vi "Extract core 2D array.vi"(8 "error in (no error)":errorcluster, 10 "Core extraction size":i32=25, 11 "Image Pixels (I16)":i16[][](array[numeric])=array512x512[262144 elements]) -> (0 "error out":errorcluster, 3 "subarray":i16[][](array[numeric]))   [LabVIEW 2020]
panel:
  out "dim2_length":i32
  out "dim2_start":i32
  out "dim1_length":i32
  out "dim1_start":i32
  out "output variable 6":dbl
  out "output variable 5":dbl
  out "output variable 4":dbl
  out "output variable 3":dbl
  out "output variable 2":i32
  out "output variable":i32
  out "size(s)":i32[](array[numeric])
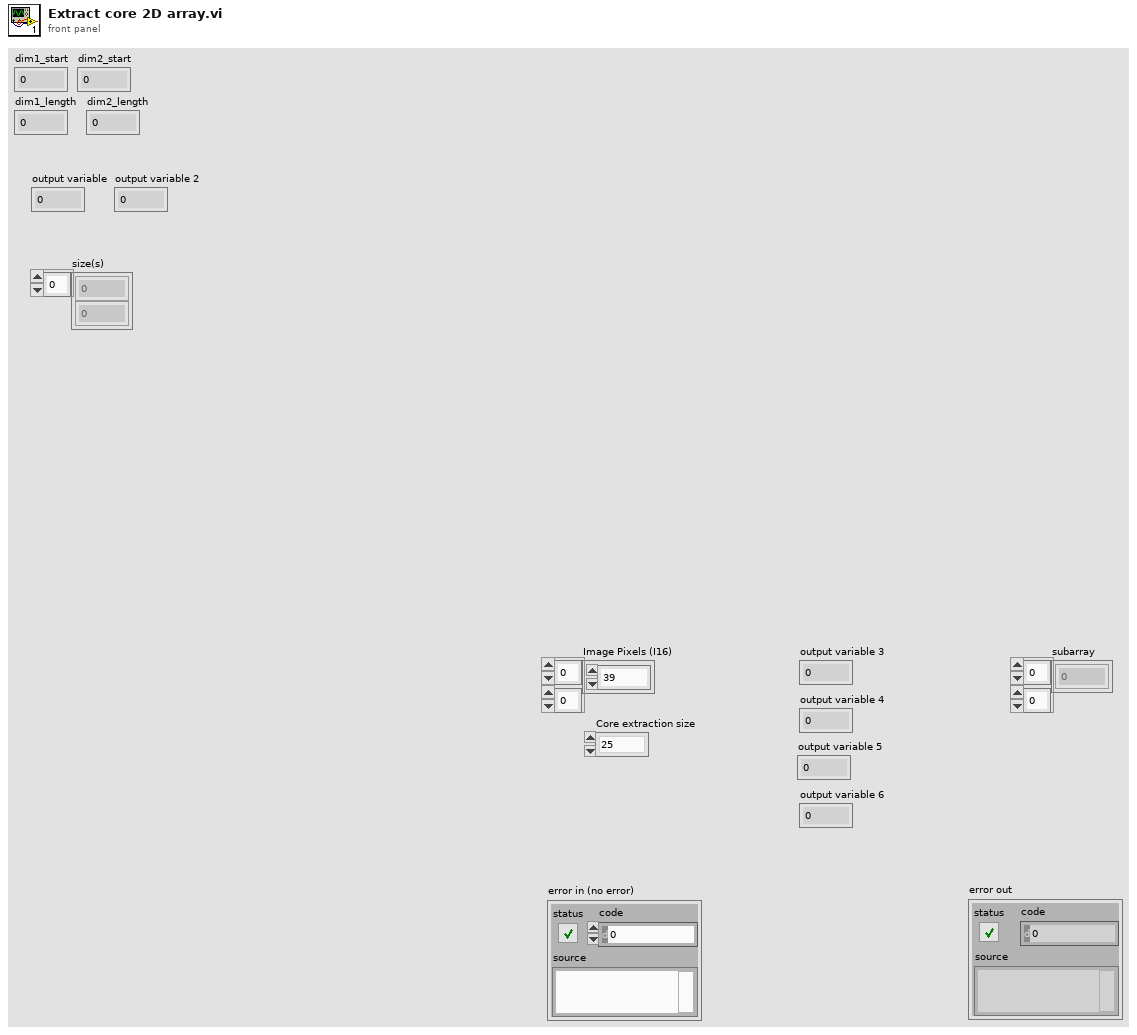
[diagram p1: front panel]
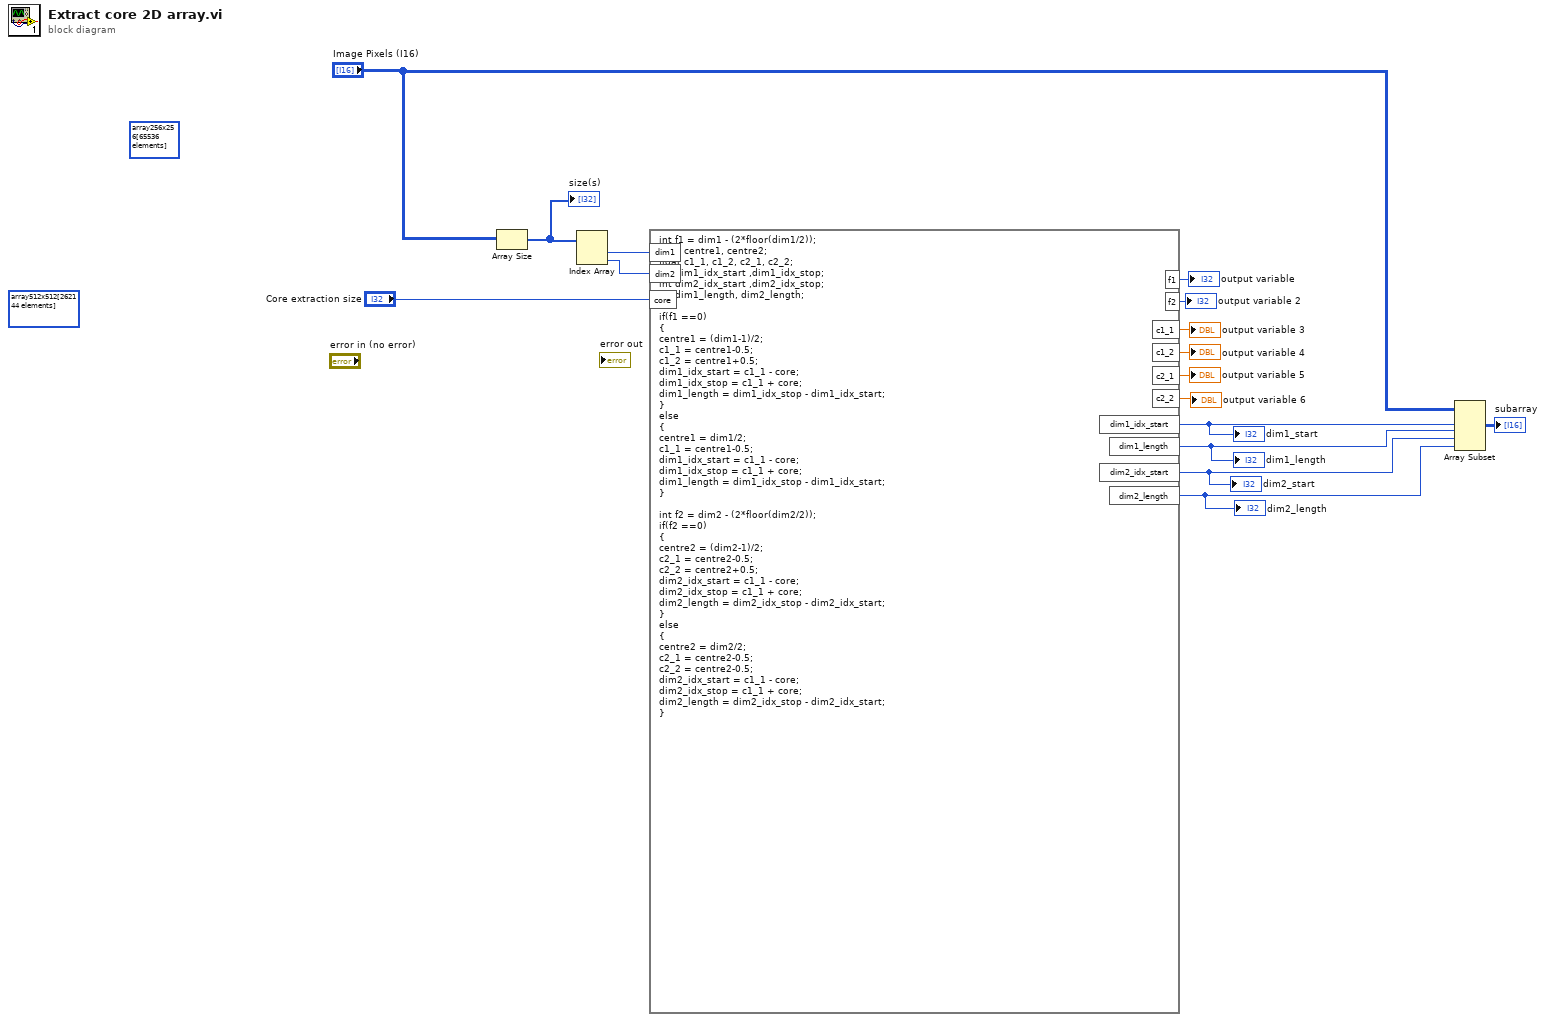
[diagram p0: block diagram]
diagram:
  (unwired) i16[][] array256x256[65536 elements] ("Image Pixels (I16)")
  (unwired) i16[][] array512x512[262144 elements] ("Intensity Graph 3")
  n1 = Array Size(array="Image Pixels (I16)") -> (size(s)=w16:i32[])
  "size(s)" <- w16
  n2 = Index Array(array=w16) -> (element #1=w15:i32, element #2=w14:i32)  [unwired: 2 in]
  n3 = formula code="int f1 = dim1 - (2*floor(dim1/2));\nfloat centre1, centre2;\nfloat c1_1, c1_2, c2_1, c2_2;\nint dim1_idx_start ,dim1_idx_stop;\nint dim2_idx_start ,dim2_idx_stop;\nint dim1_length, dim2_length;\n\nif(f1 ==0)\n{\ncentre1 = (dim1-1)/2;\nc1_1 = centre1-0.5;\nc1_2 = centre1+0.5;\ndim1_idx_start = c1_1 - core;\ndim1_idx_stop = c1_1 + core;\ndim1_length = dim1_idx_stop - dim1_idx_start;\n}\nelse\n{\ncentre1 = dim1/2;\nc1_1 = centre1-0.5;\ndim1_idx_start = c1_1 - core;\ndim1_idx_stop = c1_1 + core;\ndim1_length = dim1_idx_stop - dim1_idx_start;\n}\n\nint f2 = dim2 - (2*floor(dim2/2));\nif(f2 ==0)\n{\ncentre2 = (dim2-1)/2;\nc2_1 = centre2-0.5;\nc2_2 = centre2+0.5;\ndim2_idx_start = c1_1 - core;\ndim2_idx_stop = c1_1 + core;\ndim2_length = dim2_idx_stop - dim2_idx_start;\n}\nelse\n{\ncentre2 = dim2/2;\nc2_1 = centre2-0.5; \nc2_2 = centre2-0.5;\ndim2_idx_start = c1_1 - core;\ndim2_idx_stop = c1_1 + core;\ndim2_length = dim2_idx_stop - dim2_idx_start;\n}"("dim1"=w15, "dim2"=w14, "core"="Core extraction size") -> ("f1"=→"output variable":i32, "f2"=→"output variable 2":i32, "c1_1"=→"output variable 3":dbl, "c1_2"=→"output variable 4":dbl, "c2_1"=→"output variable 5":dbl, "c2_2"=→"output variable 6":dbl, "dim1_idx_start"=w6:i32, "dim1_length"=w5:i32, "dim2_idx_start"=w4:i32, "dim2_length"=w3:i32)
  "dim1_start" <- w6
  "dim1_length" <- w5
  "dim2_start" <- w4
  "dim2_length" <- w3
  n4 = Array Subset(array="Image Pixels (I16)", index (row)=w6, length (row)=w5, index (col)=w4, length (col)=w3) -> (→"subarray":i16[][])
